vi "subvi_45_deg_flag.vi"(6 "file (use dialog)":path, 8 "Directions":cluster{"Analyser 1":bool, "Analyser 2":bool}, 9 "Analysers Moving?":T1, 11 "Current Angles":cluster{"Analyser 1":i32, "Analyser 2":i32}) -> (1 "Found Home?":cluster{"Analyser 1":bool, "Analyser 2":bool}, 3 "New Current Angles":cluster{"Numeric Control":i32, "Analyser 2":i32})   [LabVIEW 2014]
doc: "Set Analysers Moving? to a True for one analyser to move.\nThe Direction is written to the motor.\nThe analyser specified is stepped until the 45 degree flag is hit. If the flag is hit then 45 degrees is written to the file and returned as a Current Angle. The Found Home? flag is also returned as True if the 45 degree flag is hit."
panel:
  # "INPUTS"
  # "False = +ve direction\nTrue = -ve direction"
  # "OUTPUTS"
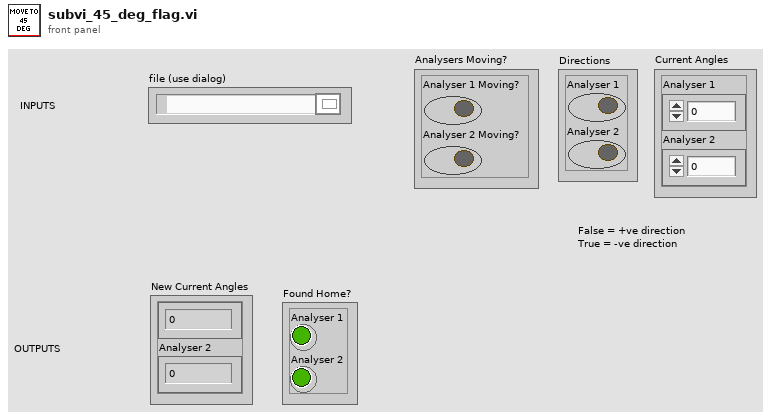
[diagram p1: front panel]
types:
  T1 = cluster{"Analyser 1 Moving?":bool, "Analyser 2 Moving?":bool}
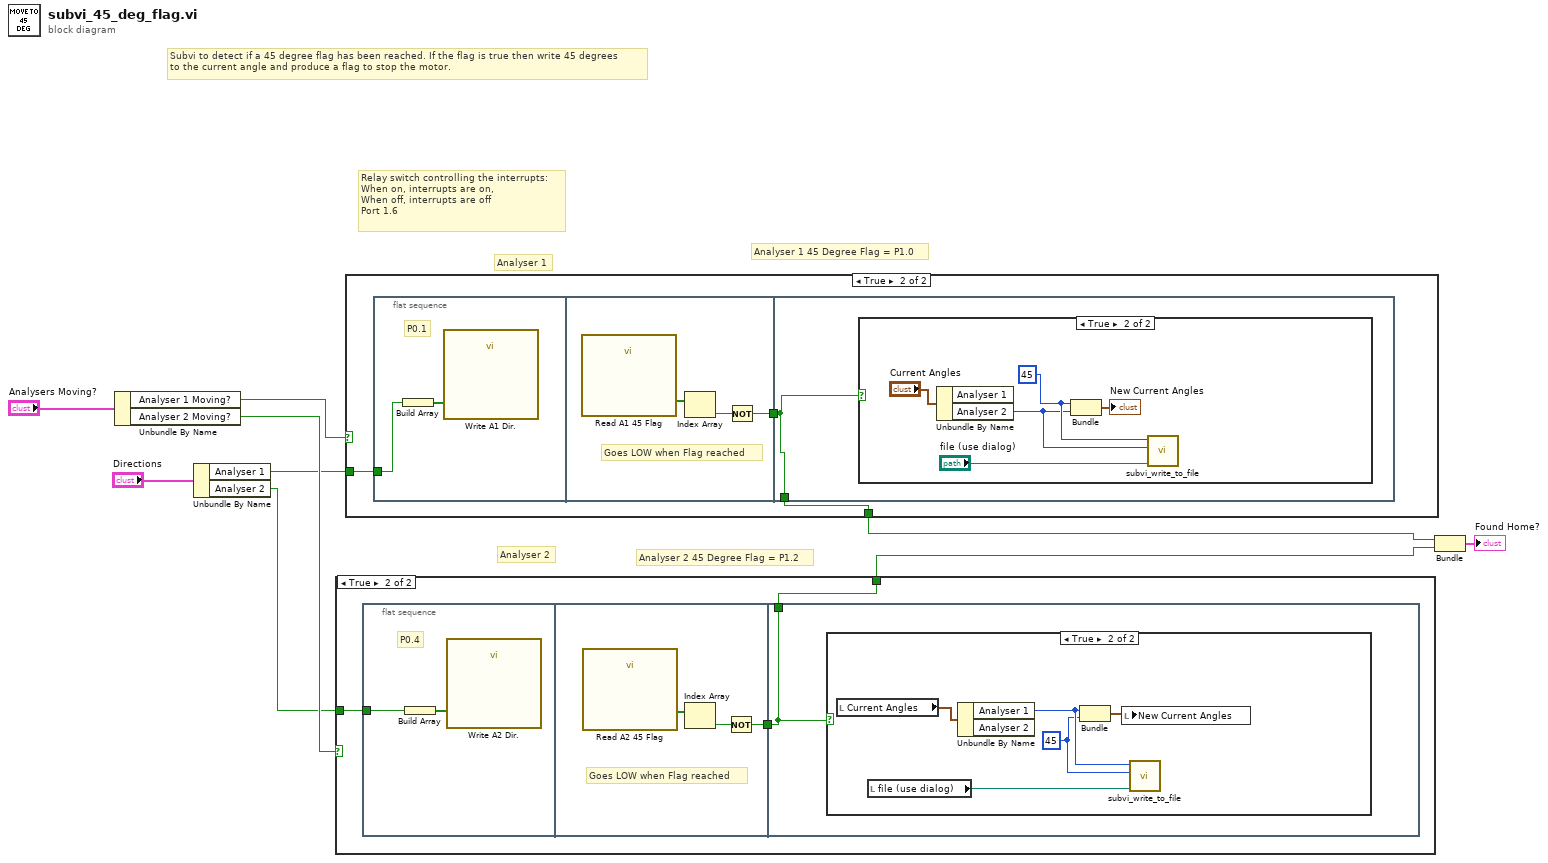
[diagram p0: block diagram]
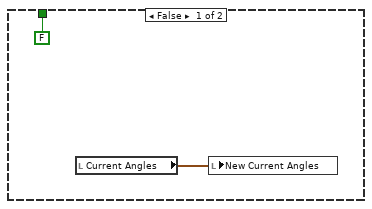
[diagram p2: hidden frame]
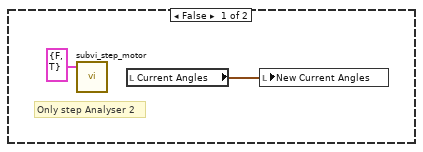
[diagram p3: hidden frame]
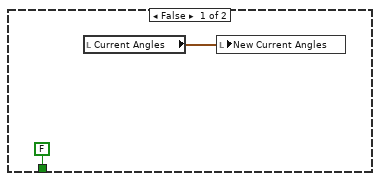
[diagram p4: hidden frame]
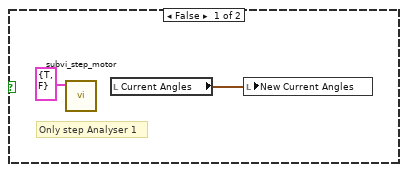
[diagram p5: hidden frame]
diagram:
  # "Analyser 2 45 Degree Flag = P1.2"
  # "Analyser 1 45 Degree Flag = P1.0"
  # "Analyser 2"
  # "Analyser 1"
  # "Relay switch controlling the interrupts:\nWhen on, interrupts are on,\nWhen off, interrupts are off\nPort 1.6"
  # "Subvi to detect if a 45 degree flag has been reached. If the flag is true then write 45 degrees\nto the current angle and produce a flag to stop the motor."
  n1 = Unbundle By Name("Analysers Moving?") -> ("Analyser 1 Moving?"=w7:bool, "Analyser 2 Moving?"=w6:bool)
  n2 = Unbundle By Name("Directions") -> ("Analyser 1"=w2:bool, "Analyser 2"=w1:bool)
  n3 = case shown="True" w6 {
    tunnel: [FALSE ("Boolean") w14] -> w3
    tunnel: w1 -> [_ w12]
    frame False {
      n4 = local read "Current Angles"() -> (w10:cluster{"Analyser 1":i32, "Analyser 2":i32})
      n5 = local write "New Current Angles"(w10) -> ()
    }
    frame True {
      n6 = flat-sequence {
        tunnel: w12 -> [w15]
        tunnel: [w17] -> w13
        tunnel: [w20] -> w14
        tunnel: w13 -> [w20]
        frame #0 {
          # "P0.4"
          n7 = Build Array(w15) -> (w16:bool[])
          n8 = call "Write A2 Dir."("data"=w16) -> ()  [unwired: 17 in, 2 out]
        }
        frame #1 {
          # "Goes LOW when Flag reached"
          n9 = call "Read A2 45 Flag"() -> ("data"=w19:bool[])  [unwired: 17 in, 2 out]
          n10 = Index Array(array=w19) -> (element=w18:bool)  [unwired: 1 in]
          n11 = Not(x=w18) -> (.not. x?=w17:bool)
        }
        frame #2 {
          n12 = case shown="True" w20 {
            frame False {
              # "Only step Analyser 2"
              n13 = call "subvi_step_motor.vi"("Write to Motor?"=cluster{"Analyser 1":bool, "Analyser 2":bool} {"Analyser 1"=FALSE, "Analyser 2"=TRUE}) -> ()  [unwired: 11 in]
              n14 = local read "Current Angles"() -> (w21:cluster{"Analyser 1":i32, "Analyser 2":i32})
              n15 = local write "New Current Angles"(w21) -> ()
            }
            frame True {
              w24 = 45
              n16 = local read "Current Angles"() -> (w27:cluster{"Analyser 1":i32, "Analyser 2":i32})
              n17 = local read "file (use dialog)"() -> (w23:path)
              n18 = Unbundle By Name(w27) -> ("Analyser 1"=w25:i32)  [unwired: 1 out]
              n19 = Bundle("Analyser 1"=w25, w24) -> (w26:cluster{"Analyser 1":i32, i32})  [unwired: 1 in]
              n20 = local write "New Current Angles"(w26) -> ()
              n21 = call "subvi_write_to_file.vi"("file (use dialog) in"=w23, "Analyser2"=w24, "Analyser 1"=w25) -> ()  [unwired: 9 in]
            }
          }
        }
      }
    }
  }
  n22 = case shown="True" w7 {
    tunnel: [FALSE ("Boolean") w31] -> w4
    tunnel: w2 -> [_ w30]
    frame False {
      n23 = local read "Current Angles"() -> (w28:cluster{"Analyser 1":i32, "Analyser 2":i32})
      n24 = local write "New Current Angles"(w28) -> ()
    }
    frame True {
      n25 = flat-sequence {
        tunnel: w30 -> [w33]
        tunnel: [w35] -> w32
        tunnel: w32 -> [w38]
        tunnel: [w38] -> w31
        frame #0 {
          # "P0.1"
          n26 = Build Array(w33) -> (w34:bool[])
          n27 = call "Write A1 Dir."("data"=w34) -> ()  [unwired: 17 in, 2 out]
        }
        frame #1 {
          # "Goes LOW when Flag reached"
          n28 = call "Read A1 45 Flag"() -> ("data"=w37:bool[])  [unwired: 17 in, 2 out]
          n29 = Index Array(array=w37) -> (element=w36:bool)  [unwired: 1 in]
          n30 = Not(x=w36) -> (.not. x?=w35:bool)
        }
        frame #2 {
          n31 = case shown="True" w38 {
            frame False {
              # "Only step Analyser 1"
              n32 = call "subvi_step_motor.vi"("Write to Motor?"=cluster{"Analyser 1":bool, "Analyser 2":bool} {"Analyser 1"=TRUE, "Analyser 2"=FALSE}) -> ()  [unwired: 11 in]
              n33 = local read "Current Angles"() -> (w39:cluster{"Analyser 1":i32, "Analyser 2":i32})
              n34 = local write "New Current Angles"(w39) -> ()
            }
            frame True {
              w42 = 45
              n35 = Unbundle By Name("Current Angles") -> ("Analyser 2"=w41:i32)  [unwired: 1 out]
              n36 = Bundle(w42, "Analyser 2"=w41) -> (→"New Current Angles":cluster{i32, "Analyser 2":i32})  [unwired: 1 in]
              n37 = call "subvi_write_to_file.vi"("file (use dialog) in"="file (use dialog)", "Analyser2"=w41, "Analyser 1"=w42) -> ()  [unwired: 9 in]
            }
          }
        }
      }
    }
  }
  n38 = Bundle("Boolean"=w4, "Boolean"=w3) -> (→"Found Home?":cluster{"Boolean":bool, "Boolean":bool})  [unwired: 1 in]
